vi "regex in string.vi"(0 "string":string, 1 "regular expression":string="[^a-zA-Z0-9]", 2 "Error String":string, 11 "error in (no error)":errorcluster) -> (4 "Error String Out":string, 8 "reg ex is in the string?":bool, 15 "error out":errorcluster)   [LabVIEW 2012]
uses:
  <vilib>/regexp/Match Regular Expression.xnode
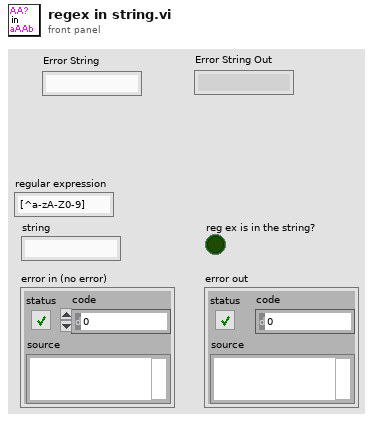
[diagram p1: front panel]
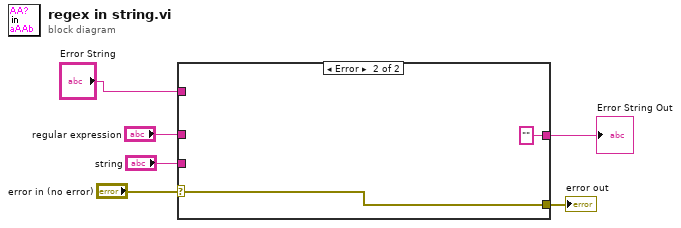
[diagram p0: block diagram]
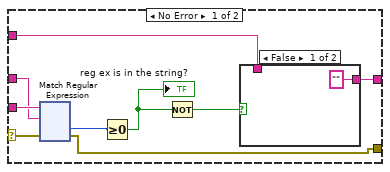
[diagram p2: hidden frame]
diagram:
  n1 = case shown="Error" "error in (no error)" {
    selector: "error in (no error)" -> [w9 w130]
    tunnel: "string" -> [w15 _]
    tunnel: "regular expression" -> [w11 _]
    tunnel: "Error String" -> [w10 _]
    tunnel: [w7 w130] -> w4
    tunnel: [w8 "" ("String")] -> w1
    frame No Error {
      n2 = xnode "Match Regular Expression"("input string"=w15, "regular expression"=w11, "error in"=w9) -> ("offset past match"=w12:i32, "error out"=w7:errorcluster)  [unwired: 3 in, 3 out]
      n3 = Greater Or Equal To 0?(x=w12) -> (x >= 0?=w14:bool)
      "reg ex is in the string?" <- w14
      n4 = Not(x=w14) -> (.not. x?=w13:bool)
      n5 = case shown="False" w13 {
        tunnel: w10 -> [_ w17]
        tunnel: ["" ("String") w17] -> w8
        frame False {
        }
        frame True {
        }
      }
    }
    frame Error {
    }
  }
  "error out" <- w4
  "Error String Out" <- w1
